vi "SMART_ScanBoxB_Loopready.vi"(10 "Smart预处理":string[][](array[string]), 11 "String数据源":string) -> ()   [LabVIEW 2017]
uses:
  <vilib>/Utility/miscctls.llb/LVPointTypeDef.ctl
panel:
  in  "Smart发送预处理btn":bool
  out "预处理后文本":string
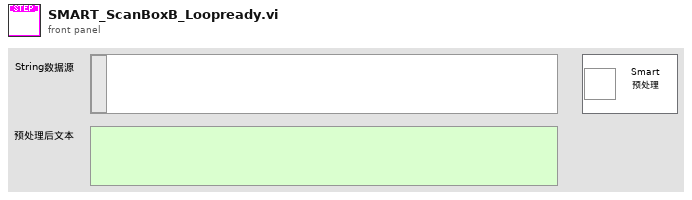
[diagram p1: front panel]
types:
  T1 = typedef "LVPointTypeDef.ctl" = cluster{"Horizontal":i16, "Vertical":i16}
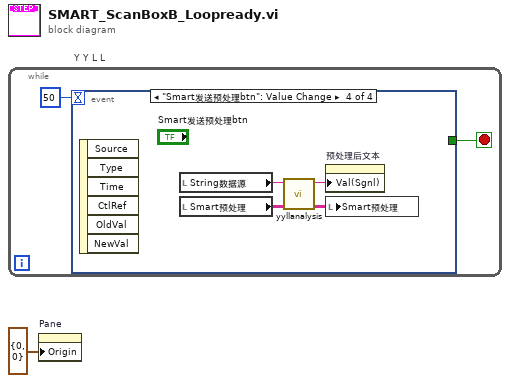
[diagram p0: block diagram]
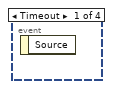
[diagram p2: hidden frame]
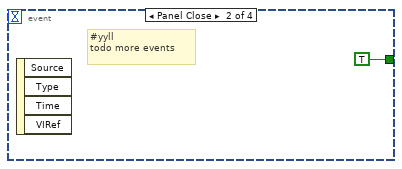
[diagram p3: hidden frame]
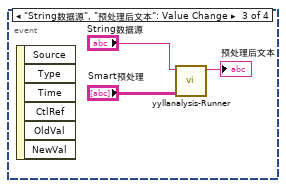
[diagram p4: hidden frame]
diagram:
  # "Y Y L L"
  n1 = while {
    stop <- w2 stop-if-true
    n2 = event shown="[3] \"Smart发送预处理btn\": Value Change" {
      selector: _ -> [_ _ _ _]
      dyn-events: _ -> [_ _ _ _]
      timeout: 50 -> [_ _ _ _]
      tunnel: [_ TRUE ("Discard?") _ _] -> w2
      event Timeout {
        n3 = event-data() -> ()  [unwired: 1 in, 1 out]
      }
      event Panel Close {
        # "#yyll\ntodo more events"
        n4 = event-data() -> ()  [unwired: 1 in, 4 out]
      }
      event "String数据源", "预处理后文本": Value Change {
        n5 = event-data() -> ()  [unwired: 1 in, 6 out]
        n6 = call "yyllanalysis-Runner.vi"("inputs"="Smart预处理", "String in"="String数据源") -> ("String out"=→"预处理后文本":string)  [unwired: 8 in, 1 out]
      }
      event "Smart发送预处理btn": Value Change {
        n7 = event-data() -> ()  [unwired: 1 in, 6 out]
        n8 = local read "String数据源"() -> (w8:string)
        n9 = local read "Smart预处理"() -> (w11:string[][])
        n10 = call "yyllanalysis.vi"("Datain"=w11, "StringIN"=w8) -> ("Dataout"=w10:string[][], "StringOUT"=w9:string)  [unwired: 8 in]
        n11 = property on="预处理后文本" class="Str"("Val(Sgnl)"=w9) -> ()  [unwired: 2 in, 2 out]
        n12 = local write "Smart预处理"(w10) -> ()
      }
    }
  }
  n13 = property on="Pane" class="Pane"("Origin"=T1 {"Horizontal"=0, "Vertical"=0}) -> ()  [unwired: 2 in, 2 out]
